vi "Set FIFOs.vi"(8 "error in (no error)":errorcluster, 9 "Output":refnum<k21>, 10 "Input":refnum<k21>, 11 "TestMPU in":refnum<class "TestMPU.lvclass">) -> (0 "error out":errorcluster, 3 "TestMPU out":refnum<class "TestMPU.lvclass">)   [LabVIEW 2018, in "TestMPU.lvclass"]
uses:
  TestMPU.lvclass
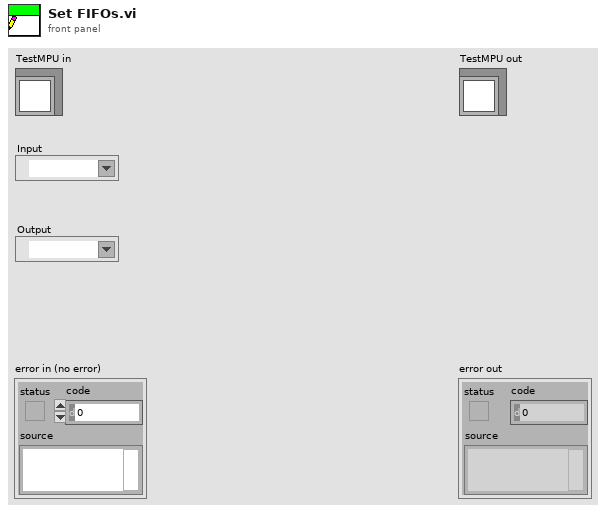
[diagram p1: front panel]
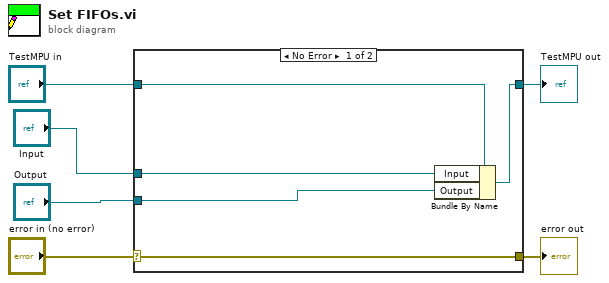
[diagram p0: block diagram]
diagram:
  n1 = case shown="No Error" "error in (no error)" {
    selector: "error in (no error)" -> [w11 w12]
    tunnel: [w11 w12] -> w5
    tunnel: [w9 w13] -> w3
    tunnel: "TestMPU in" -> [w10 w13]
    tunnel: "Input" -> [w8 _]
    tunnel: "Output" -> [w7 _]
    frame No Error {
      n2 = Bundle By Name(cluster=w10, "Input"=w8, "Output"=w7) -> (w9:refnum<class "TestMPU.lvclass">)
    }
    frame Error {
    }
  }
  "error out" <- w5
  "TestMPU out" <- w3
